vi "Server ATM machine.vi"() -> ()   [LabVIEW 2020]
uses:
  Sub VIs/Enum (Server).ctl
  <vilib>/Utility/file.llb/Read Delimited Spreadsheet (string).vi
  <vilib>/Utility/file.llb/Write Delimited Spreadsheet (string).vi
panel:
  out "Row Index":i32
  out "Account No from client":string
  out "String sent back to client":string
  out "ArraySize":i32
  in  "Server ATM Machine":enum32{"Page 1"}(tab)
  in  "Register Button":bool
  in  "User Table":string[][](table)
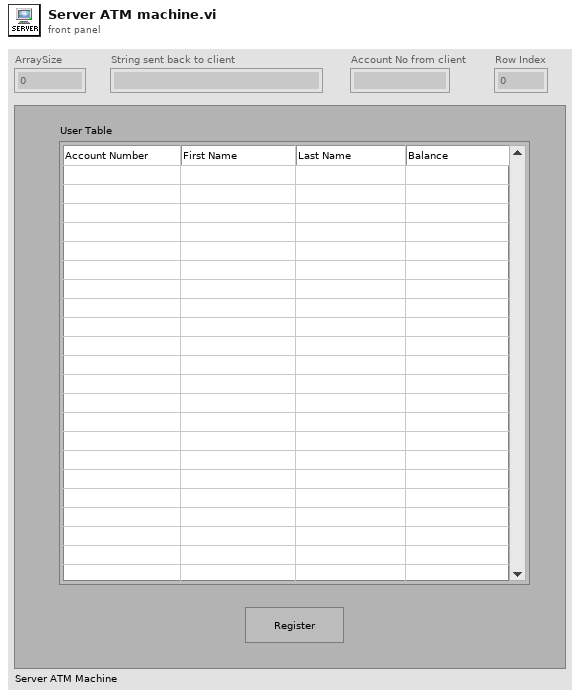
[diagram p1: front panel]
types:
  T1 = typedef "Enum (Server).ctl" = enum16{"Verify", "Update File"}
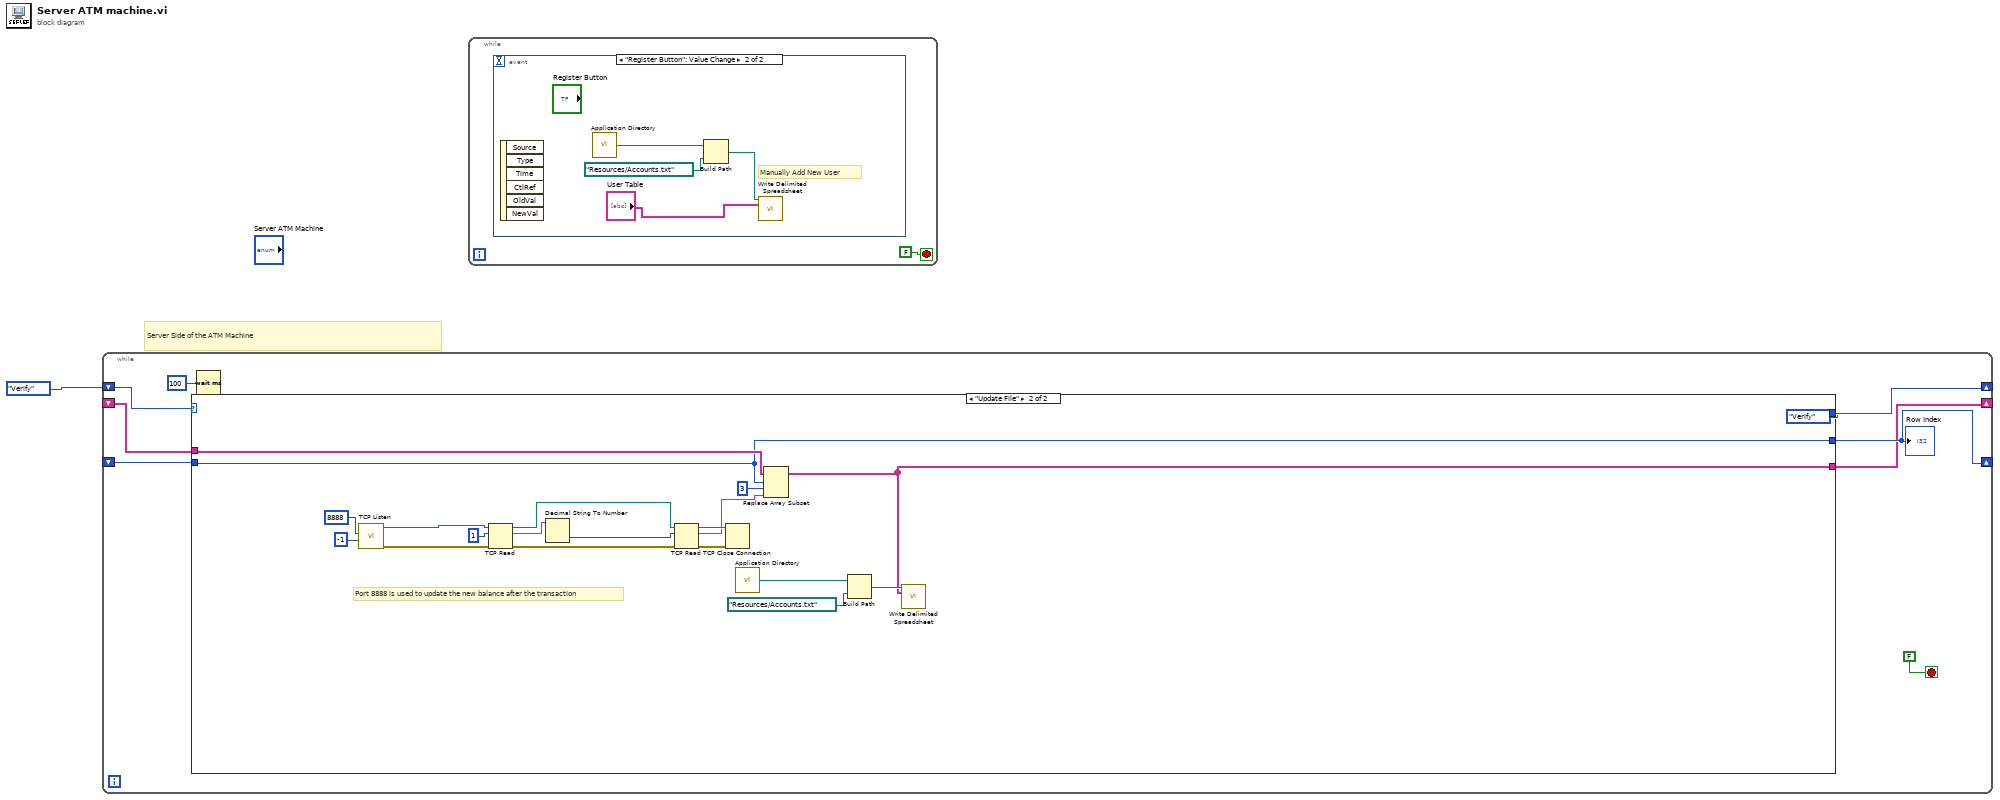
[diagram p0: block diagram]
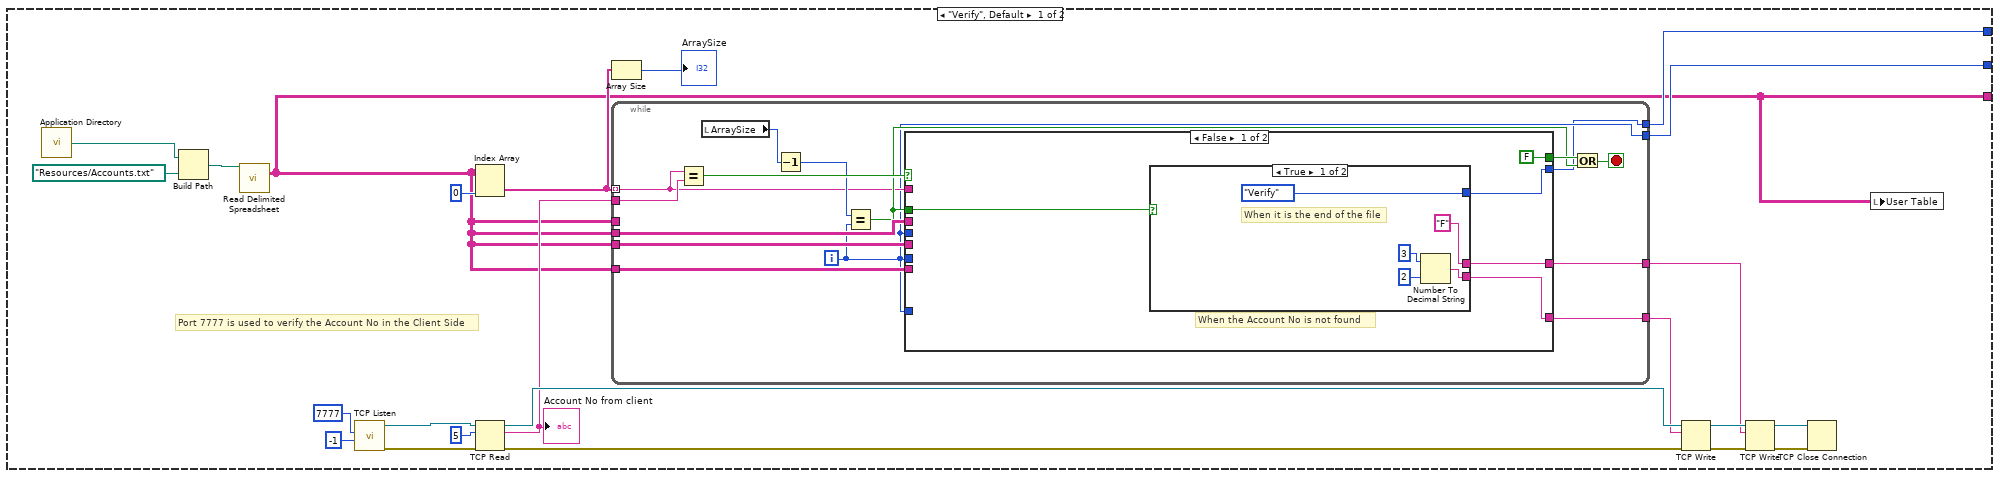
[diagram p2: hidden frame]
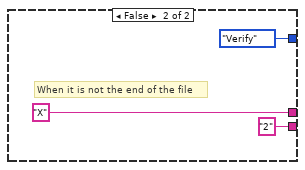
[diagram p3: hidden frame]
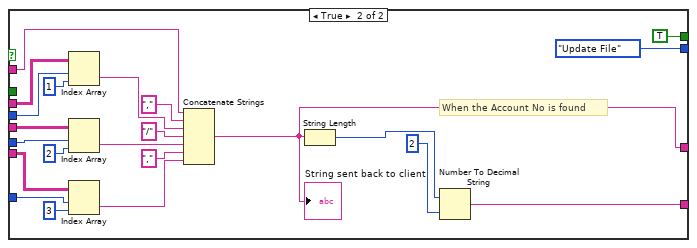
[diagram p4: hidden frame]
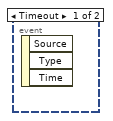
[diagram p5: hidden frame]
diagram:
  # "Server Side of the ATM Machine"
  n1 = while {
    shift-right: [w7] -> _
    shift-left: Enum_(Server)."Verify" -> [w8]
    shift-right: [w6] -> _
    shift-left: _ -> [w5]
    shift-right: [w4] -> _
    shift-left: _ -> [w3]
    stop <- FALSE stop-if-true
    n2 = case shown="\"Update File\"" w8 {
      tunnel: [w12 w83] -> w6
      tunnel: [w11 Enum_(Server)."Verify"] -> w7
      tunnel: w5 -> [_ w83]
      tunnel: [w10 w85] -> w4
      tunnel: w3 -> [_ w84]
      frame "Verify", Default {
        # "Port 7777 is used to verify the Account No in the Client Side"
        n3 = call <vilib>:"Application Directory.vi"() -> ("Application Directory"=w13:path)
        n4 = Build Path(base path=w13, name or relative path=path "Resources/Accounts.txt") -> (appended path=w31:path)
        n5 = call-poly <vilib>:"Read Delimited Spreadsheet.vi"("file path (dialog if empty)"=w31) -> ("all rows"=w10:string[][])  [unwired: 9 in, 5 out]
        n6 = call <vilib>:"TCP Listen.vi"("timeout ms (wait forever: -1)"=-1, "port"=u16 7777 ("remote port or service name")) -> ("error out"=w19:errorcluster, "connection ID"=w28:refnum<k5>)  [unwired: 5 in, 3 out]
        n7 = Index Array "Index Array"(array=w10, index (col)=0 ("disabled index (col)")) -> (element=w22:string[])  [unwired: 1 in]
        n8 = TCP Read(connection ID=w28, bytes to read=5, error in (no error)=w19) -> (connection ID out=w25:refnum<k5>, data out=w24:string, error out=w20:errorcluster)  [unwired: 2 in]
        "Account No from client" <- w24
        n9 = Array Size(array=w22) -> (size(s)=→"ArraySize":i32)
        n10 = while {
          tunnel: w24 -> [w46]
          tunnel: w22 -> [w35] mode=indexing
          tunnel: w10 -> [_]
          tunnel: w10 -> [w45]
          tunnel: w10 -> [w44]
          tunnel: w10 -> [w43]
          tunnel: [w42] -> w23
          tunnel: [w41] -> w14
          tunnel: [w34] -> w12
          tunnel: [w33] -> w11
          i -> [w34]
          stop <- w37 stop-if-true
          n11 = Equal?(x=w35, y=w46) -> (x = y?=w47:bool)
          n12 = local read "ArraySize"() -> (w40:i32)
          n13 = Decrement(x=w40) -> (x-1=w39:i32)
          n14 = Equal?(x=w39, y=w34) -> (x = y?=w36:bool)
          n15 = case shown="False" w47 {
            tunnel: [FALSE TRUE] -> w38
            tunnel: w45 -> [_ w80]
            tunnel: w34 -> [_ w79]
            tunnel: w44 -> [_ w75]
            tunnel: w34 -> [_ w74]
            tunnel: w34 -> [_ w71]
            tunnel: w43 -> [_ w70]
            tunnel: [w51 w64] -> w42
            tunnel: [w50 w63] -> w41
            tunnel: w36 -> [w49 _]
            tunnel: w35 -> [_ w62]
            tunnel: [w48 Enum_(Server)."Update File"] -> w33
            frame False {
              # "When the Account No is not found"
              n16 = case shown="True" w49 {
                tunnel: [w56 "2"] -> w51
                tunnel: ["F" "X"] -> w50
                tunnel: [Enum_(Server)."Verify" Enum_(Server)."Verify"] -> w48
                frame True {
                  # "When it is the end of the file"
                  n17 = Number To Decimal String(number=3, width (-)=i16 2) -> (decimal integer string=w56:string)
                }
                frame False {
                  # "When it is not the end of the file"
                }
              }
            }
            frame True {
              # "When the Account No is found"
              n18 = Index Array "Index Array"(array=w80, index (row)=w79, index (col)=1 ("disabled index (col)")) -> (element=w77:string)
              n19 = Index Array "Index Array"(array=w75, index (row)=w74, index (col)=2 ("disabled index (col)")) -> (element=w69:string)
              n20 = Index Array "Index Array"(array=w70, index (row)=w71, index (col)=3) -> (element=w67:string)
              n21 = Concatenate Strings "Concatenate Strings"(w62, "," ("string"), w77, "/" ("string"), w69, "," ("string"), w67) -> (w63:string)
              "String sent back to client" <- w63
              n22 = String Length(string=w63) -> (length=w66:i32)
              n23 = Number To Decimal String(number=w66, width (-)=i16 2) -> (decimal integer string=w64:string)
            }
          }
          n24 = Or(x=w38, y=w36) -> (x .or. y?=w37:bool)
        }
        n25 = TCP Write(connection ID=w25, data in=w23, error in (no error)=w20) -> (connection ID out=w18:refnum<k5>, error out=w17:errorcluster)  [unwired: 1 in, 1 out]
        n26 = TCP Write(connection ID=w18, data in=w14, error in (no error)=w17) -> (connection ID out=w15:refnum<k5>, error out=w16:errorcluster)  [unwired: 1 in, 1 out]
        n27 = TCP Close Connection(connection ID=w15, error in (no error)=w16) -> ()  [unwired: 1 in, 2 out]
        n28 = local write "User Table"(w10) -> ()
      }
      frame "Update File" {
        # "Port 8888 is used to update the new balance after the transaction"
        n29 = call <vilib>:"TCP Listen.vi"("timeout ms (wait forever: -1)"=-1, "port"=u16 8888) -> ("error out"=w99:errorcluster, "connection ID"=w102:refnum<k5>)  [unwired: 5 in, 3 out]
        n30 = TCP Read(connection ID=w102, bytes to read=1, error in (no error)=w99) -> (connection ID out=w101:refnum<k5>, data out=w96:string, error out=w98:errorcluster)  [unwired: 2 in]
        n31 = Decimal String To Number(string=w96) -> (number=w95:i32)  [unwired: 2 in, 1 out]
        n32 = TCP Read(connection ID=w101, bytes to read=w95, error in (no error)=w98) -> (connection ID out=w100:refnum<k5>, data out=w94:string, error out=w97:errorcluster)  [unwired: 2 in]
        n33 = TCP Close Connection(connection ID=w100, error in (no error)=w97) -> ()  [unwired: 1 in, 2 out]
        n34 = call <vilib>:"Application Directory.vi"() -> ("Application Directory"=w92:path)
        n35 = Replace Array Subset "Replace Array Subset"(array=w84, new element=w94, index (row)=w83, index (col)=3 ("disabled index (col)")) -> (w85:string[][])
        n36 = Build Path(base path=w92, name or relative path=path "Resources/Accounts.txt") -> (appended path=w93:path)
        n37 = call-poly <vilib>:"Write Delimited Spreadsheet.vi"("file path (dialog if empty)"=w93, "2D data"=w85) -> ()  [unwired: 12 in, 2 out]
      }
    }
    "Row Index" <- w6
    n38 = Wait (ms)(milliseconds to wait=u32 100) -> ()  [unwired: 1 out]
  }
  n39 = while {
    stop <- FALSE stop-if-true
    n40 = event shown="[1] \"Register Button\": Value Change" {
      selector: _ -> [_ _]
      dyn-events: _ -> [_ _]
      timeout: _ -> [_ _]
      event Timeout {
        n41 = event-data() -> ()  [unwired: 1 in, 3 out]
      }
      event "Register Button": Value Change {
        # "Manually Add New User"
        n42 = event-data() -> ()  [unwired: 1 in, 6 out]
        n43 = call <vilib>:"Application Directory.vi"() -> ("Application Directory"=w107:path)
        n44 = Build Path(base path=w107, name or relative path=path "Resources/Accounts.txt") -> (appended path=w106:path)
        n45 = call-poly <vilib>:"Write Delimited Spreadsheet.vi"("file path (dialog if empty)"=w106, "2D data"="User Table") -> ()  [unwired: 12 in, 2 out]
      }
    }
  }
